vi "Create Differential Steering Frame.vi"(8 "error in (no error)":errorcluster, 10 "wheel separation":dbl, 11 "wheels":T1) -> (0 "error out":errorcluster, 3 "differential steering frame out":refnum<class "NI_Robotics_Differential Steering Frame.lvclass">)   [LabVIEW 2017, in "NI_Robotics_Differential Steering Frame.lvclass"]
doc: "Creates a steering frame of the type you specify. You must manually select the polymorphic instance to use."
uses:
  <vilib>/robotics/Steering/Differential Steering Frame/NI_Robotics_Differential Steering Frame.lvclass
  c:/Program Files (x86)/National Instruments/LabVIEW 2017/vi.lib/robotics/Steering/Steering Frame/NI_Robotics_Steering Frame.lvclass
  <vilib>/robotics/Steering/Differential Steering Frame/Differential Wheel Group.ctl
  <vilib>/robotics/Steering/Fixed Wheel/NI_Robotics_Fixed Wheel.lvclass
  c:/Program Files (x86)/National Instruments/LabVIEW 2017/vi.lib/robotics/Steering/Wheel/NI_Robotics_Wheel.lvclass
  <vilib>/robotics/Steering/Wheel/Rotation Direction.ctl
  <vilib>/robotics/Steering/Wheel/NI_Robotics_Wheel.lvclass/NI_Robotics_Wheel.ctl
  <vilib>/robotics/Steering/Steering Frame/NI_Robotics_Steering Frame.lvclass/NI_Robotics_Steering Frame.ctl
  <vilib>/robotics/Steering/Differential Steering Frame/NI_Robotics_Differential Steering Frame.lvclass/NI_Robotics_Differential Steering Frame.ctl
  <vilib>/robotics/Steering/Wheel/Get Wheel Name.vi
  <vilib>/robotics/Steering/Wheel/Update Steering to Wheel Frame Transform.vi
  <vilib>/Analysis/coordinate.llb/Wrap Angle.vi
  <vilib>/Analysis/coordinate.llb/Wrap Angle (array).vi
  <vilib>/robotics/Steering/Wheel/NI_Robotics_Wheel.lvclass
  <vilib>/robotics/Steering/Steering Frame/NI_Robotics_Steering Frame.lvclass
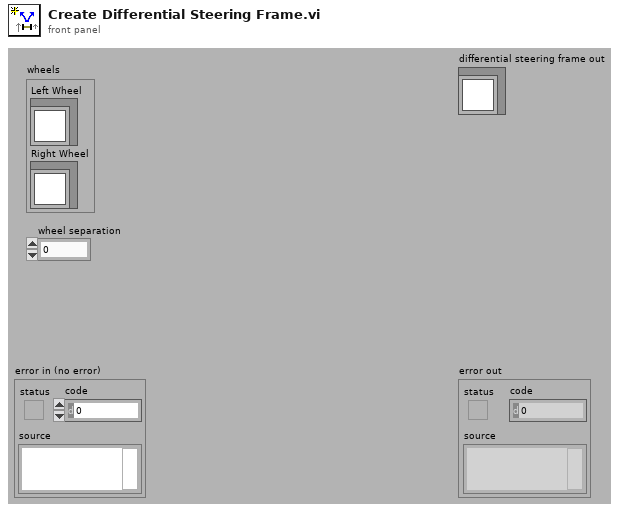
[diagram p1: front panel]
types:
  T1 = typedef "NI_Robotics_Differential Steering Frame.lvclass/Differential Wheel Group.ctl" = cluster{"Left Wheel":refnum<class "NI_Robotics_Fixed Wheel.lvclass">, "Right Wheel":refnum<class "NI_Robotics_Fixed Wheel.lvclass">}
  T2 = typedef "NI_Robotics_Wheel.lvclass/Rotation Direction.ctl" = u16
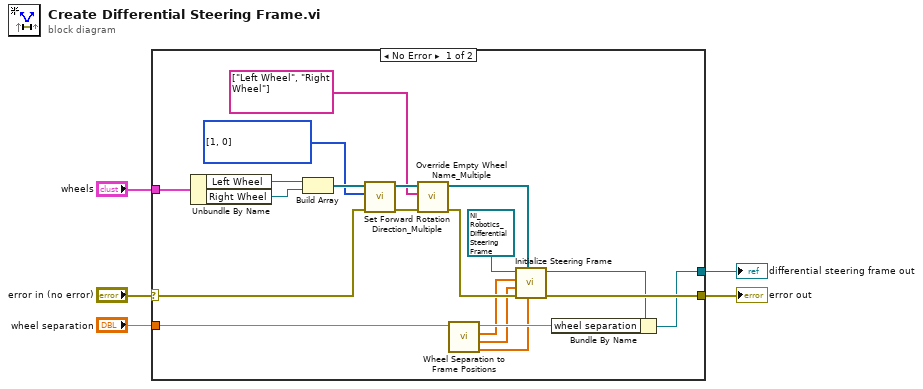
[diagram p0: block diagram]
diagram:
  n1 = case shown="No Error" "error in (no error)" {
    selector: "error in (no error)" -> [w20 w26]
    tunnel: [w24 w26] -> w4
    tunnel: [w11 _] -> w3
    tunnel: "wheel separation" -> [w10 _]
    tunnel: "wheels" -> [w23 _]
    frame No Error {
      w18 = T2[] [1, 0] items=["Clockwise", "Counterclockwise"] ("Forward Rotation Directions")
      n2 = Unbundle By Name(w23) -> ("Left Wheel"=w22:refnum<class "NI_Robotics_Fixed Wheel.lvclass">, "Right Wheel"=w21:refnum<class "NI_Robotics_Fixed Wheel.lvclass">)
      n3 = Build Array(w22, w21) -> (w19:refnum<class "NI_Robotics_Fixed Wheel.lvclass">[])
      n4 = call <vilib>:"Set Forward Rotation Direction_Multiple.vi"("error in (no error)"=w20, "forward rotation directions"=w18, "wheels in"=w19) -> ("error out"=w15:errorcluster, "wheels out"=w17:refnum<class "NI_Robotics_Wheel.lvclass">[])  [unwired: 7 in]
      n5 = call <vilib>:"Override Empty Wheel Name_Multiple.vi"("error in (no error)"=w15, "wheel names"=string[] ["Left Wheel", "Right Wheel"] ("Wheel IDs"), "wheels in"=w17) -> ("error out"=w14:errorcluster, "wheels out"=w16:refnum<class "NI_Robotics_Wheel.lvclass">[])  [unwired: 7 in]
      n6 = call <vilib>:"Wheel Separation to Frame Positions.vi"("wheel separation"=w10) -> ("wheel frame angles (rad)"=w6:dbl[], "wheel y positions"=w7:dbl[], "wheel x positions"=w8:dbl[], "coerced wheel separation"=w9:dbl)  [unwired: 6 in, 1 out]
      n7 = call <vilib>:"Initialize Steering Frame.vi"("wheel frame angles (rad)"=w6, "wheels"=w16, "error in (no error)"=w14, "wheel y positions"=w7, "wheel x positions"=w8, "steering frame in"=refnum<class "NI_Robotics_Differential Steering Frame.lvclass"> refnum ("Differential Steering Frame in")) -> ("error out"=w24:errorcluster, "steering frame out"=w12:refnum<class "NI_Robotics_Differential Steering Frame.lvclass">)  [unwired: 4 in]
      n8 = Bundle By Name(cluster=w12, "wheel separation"=w9) -> (w11:refnum<class "NI_Robotics_Differential Steering Frame.lvclass">)
    }
    frame Error {
    }
  }
  "error out" <- w4
  "differential steering frame out" <- w3
